vi "Read Config Hash.vi"(8 "error in (no error)":errorcluster, 11 "System Config Server in":refnum<class "System Config Server.lvclass">) -> (0 "error out":errorcluster, 3 "System Config Server out":refnum<class "System Config Server.lvclass">)   [LabVIEW 2020, in "Volatus.lvlib" / "System Config Server.lvclass"]
uses:
  System Config Server.lvclass
  System Config Server.lvclass/System Config Server.ctl
  <vilib>/security/Message Digest/API/NI_Message Digest API.lvlib
  <vilib>/security/Message Digest/API/Instances/Byte Array/SHA-256 Byte Array Checksum.vi
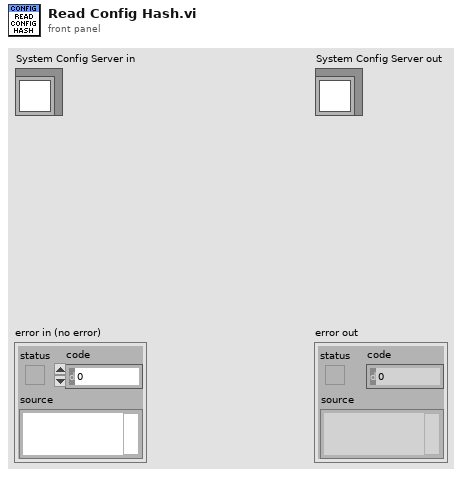
[diagram p1: front panel]
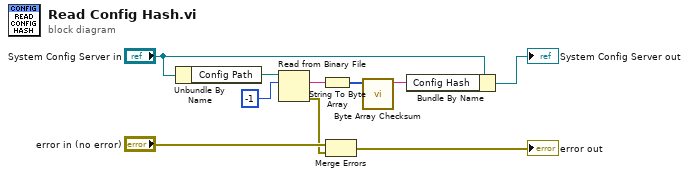
[diagram p0: block diagram]
diagram:
  n1 = Unbundle By Name("System Config Server in") -> ("Config Path"=w8:path)
  n2 = Read from Binary File(10:-1 ("count (1)"), 11:w8) -> (0:w1:errorcluster, 2:w6:string)  [unwired: 4 in, 2 out]
  n3 = String To Byte Array(string=w6) -> (unsigned byte array=w5:u8[])
  n4 = Merge Errors("error in (no error)", w1) -> (→"error out":errorcluster)
  n5 = call-poly <vilib>:"Byte Array Checksum.vi"("buffer"=w5) -> ("digest"=w3:string)  [unwired: 10 in]
  n6 = Bundle By Name(cluster="System Config Server in", "Config Hash"=w3) -> (→"System Config Server out":refnum<class "System Config Server.lvclass">)
